vi "WPI_CameraSetScaledAttr.vi"(6 "Exposure Fixup?":bool, 7 "Attr Format":string="CameraAttributes::%s::Value", 8 "error in (no error)":errorcluster, 9 "Scaled":dbl, 10 "Attr String":string, 11 "Camera Address In":string) -> (0 "error out":errorcluster, 3 "Camera Address Out":string)   [LabVIEW 2017]
doc: "This VI updates an attribute where input unit is percentage and camera parameter may be in another unit.\n\nThis software is licensed. Open the labview\\readme\\WPI Robotics Library Open Source License.txt file for more information."
uses:
  <vilib>/userdefined/High Color/IMAQdx.ctl
  <resource>/objmgr/imaqdx.rc
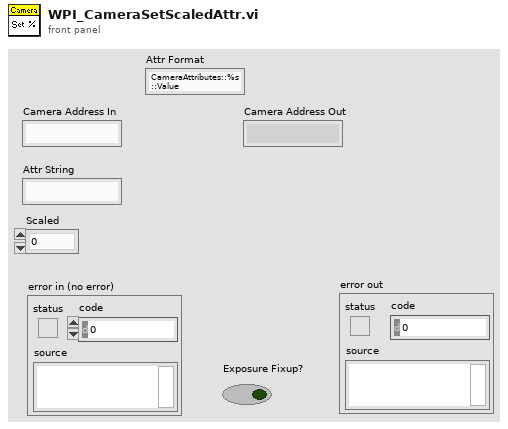
[diagram p1: front panel]
types:
  T1 = typedef "IMAQdx.ctl" = refnum<k21>
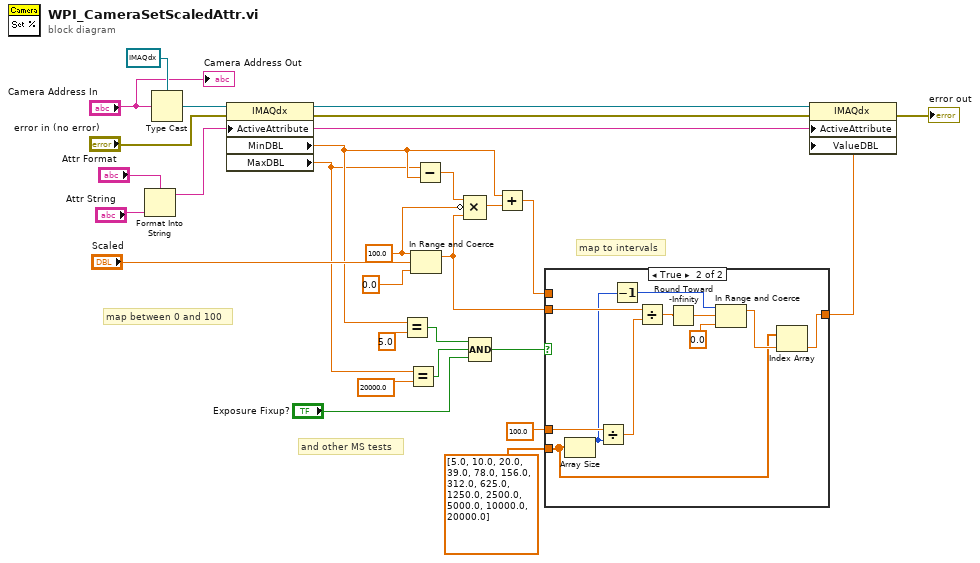
[diagram p0: block diagram]
diagram:
  w20 = 100.0
  # "map to intervals"
  # "and other MS tests"
  # "map between 0 and 100"
  n1 = Format Into String(format string="Attr Format", "Attr String") -> (resulting string=w17:string)  [unwired: 2 in, 1 out]
  n2 = Type Cast(type=T1 refnum ("Session In"), x="Camera Address In") -> (*(type *) &x=w27:T1)
  n3 = property class="IMAQdx"(reference=w27, error in="error in (no error)", "ActiveAttribute"=w17) -> (reference out=w18:T1, error out=w15:errorcluster, "MinDBL"=w13:dbl, "MaxDBL"=w10:dbl)
  n4 = Equal?(x=w13, y=5.0) -> (x = y?=w9:bool)
  n5 = Equal?(x=w10, y=20000.0) -> (x = y?=w8:bool)
  n6 = In Range and Coerce(upper limit=w20, x="Scaled", lower limit=0.0) -> (coerced(x)=w6:dbl)  [unwired: 1 out]
  n7 = Subtract(x=w10, y=w13) -> (x-y=w23:dbl)
  n8 = Compound Arithmetic op=MULTIPLY(w23, invert w20, w6) -> (w19:dbl)
  n9 = Compound Arithmetic op=AND(w9, w8, "Exposure Fixup?") -> (w7:bool)
  n10 = Add(x=w13, y=w19) -> (x+y=w3:dbl)
  n11 = case shown="True" w7 {
    tunnel: w3 -> [w29 _]
    tunnel: w6 -> [_ w40]
    tunnel: dbl[] [5.0, 10.0, 20.0, 39.0, 78.0, 156.0, 312.0, 625.0, 1250.0, 2500.0, 5000.0, 10000.0, 20000.0] -> [_ w32]
    tunnel: 100.0 -> [_ w39]
    tunnel: [w29 w38] -> w2
    frame False {
    }
    frame True {
      n12 = Array Size(array=w32) -> (size(s)=w30:i32)
      n13 = Divide(x=w39, y=w30) -> (x/y=w37:dbl)
      n14 = Decrement(x=w30) -> (x-1=w31:i32)
      n15 = Divide(x=w40, y=w37) -> (x/y=w36:dbl)
      n16 = Round Toward -Infinity(1:w36) -> (0:w35:dbl)
      n17 = In Range and Coerce(upper limit=w31, x=w35, lower limit=0.0) -> (coerced(x)=w34:dbl)  [unwired: 1 out]
      n18 = Index Array(array=w32, index=w34) -> (element=w38:dbl)
    }
  }
  n19 = property class="IMAQdx"(reference=w18, error in=w15, "ActiveAttribute"=w17, "ValueDBL"=w2) -> (error out=→"error out":errorcluster)  [unwired: 1 out]
  "Camera Address Out" <- "Camera Address In"
